vi "Get Current.vi"(8 "error in (no error)":errorcluster, 10 "chan (1)":i32=1 min=0 max=3, 11 "VISA resource name":refnum<visa-resource-name>) -> (0 "error out":errorcluster, 2 "output":i32, 3 "VISA resource name out":refnum<visa-resource-name>)   [LabVIEW 2025, in "Detector SCPI.lvlib"]
doc: "Gets supply current from different power channels to detector board\nChannel 1: 3v3 supply (INA3221-1)\nChannel 2: Heater (INA3221-2)\nChannel 3: +12V (INA3221-3)\nChannel 4: -12V Supply (IN238)"
uses:
  Detector SCPI.lvlib
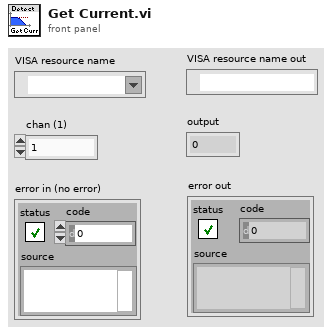
[diagram p1: front panel]
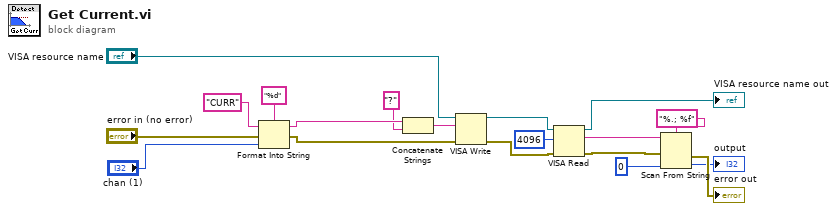
[diagram p0: block diagram]
diagram:
  n1 = Format Into String(format string="%d", initial string="CURR" ("command"), error in="error in (no error)", "chan (1)") -> (resulting string=w11:string, error out=w17:errorcluster)
  n2 = Concatenate Strings(w11, "?" ("command")) -> (w12:string)
  n3 = VISA Write(VISA resource name="VISA resource name", write buffer=w12, error in (no error)=w17) -> (VISA resource name out=w1:refnum<visa-resource-name>, error out=w13:errorcluster)  [unwired: 1 out]
  n4 = VISA Read(VISA resource name=w1, byte count=u32 4096, error in (no error)=w13) -> (VISA resource name out=→"VISA resource name out":refnum<visa-resource-name>, read buffer=w7:string, error out=w5:errorcluster)  [unwired: 1 out]
  n5 = Scan From String(format string="%.; %f", input string=w7, error in=w5, default 1=0 ("default value 1")) -> (error out=→"error out":errorcluster, output 1=→"output":i32)  [unwired: 1 in, 2 out]
